vi "Query Sweep Mode.vi"(8 "error in (no error)":errorcluster, 10 "Channel (0: Channel 1)":T2 items=["Channel 1", "Channel 2"], 11 "VISA resource name":refnum<visa-resource-name>) -> (0 "error out":errorcluster, 1 "Sweep mode (auto)":T1, 3 "VISA resource name out":refnum<visa-resource-name>)   [LabVIEW 2009, in "Tektronix AFG 3000 Series.lvlib"]
doc: "Queries the sweep mode of a Tektronix AFG 3000 series function generator; returns either auto or manual. In auto mode the AFG sweeps continuously; in manual mode, it sweeps once each time it gets a trigger."
uses:
  Tektronix AFG 3000 Series.lvlib
  controls.llb/Channel.ctl
  controls.llb/Sweep Mode.ctl
  <vilib>/Utility/error.llb/DialogType.ctl
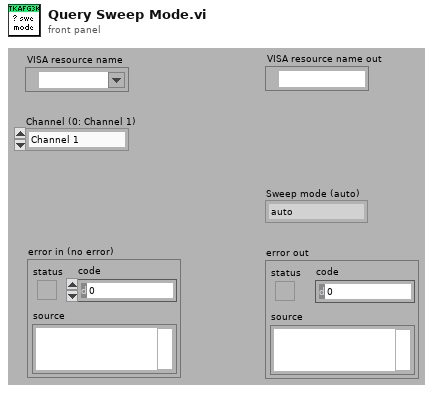
[diagram p1: front panel]
types:
  T1 = typedef "Sweep Mode.ctl" = enum16{"auto", "manual/triggered"}
  T2 = typedef "Channel.ctl" = u16
  T3 = typedef "DialogType.ctl" = u16
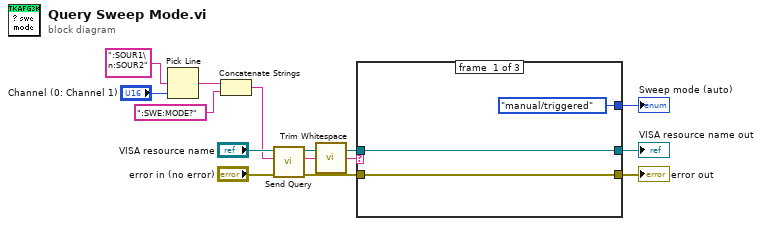
[diagram p0: block diagram]
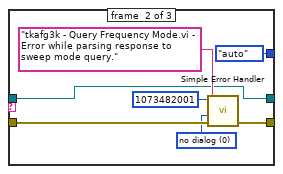
[diagram p2: hidden frame]
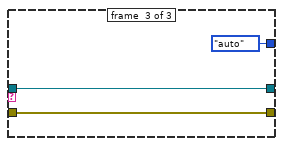
[diagram p3: hidden frame]
diagram:
  n1 = Pick Line(multi-line string=":SOUR1\n:SOUR2", line index="Channel (0: Channel 1)") -> (output string=w11:string)  [unwired: 1 out]
  n2 = Concatenate Strings(w11, ":SWE:MODE?" ("format string")) -> (w10:string)
  n3 = call "Send Query.vi"("error in (no error)"="error in (no error)", "write buffer"=w10, "VISA resource name"="VISA resource name") -> ("error out"=w7:errorcluster, "read buffer"=w3:string, "VISA resource name out"=w6:refnum<visa-resource-name>)  [unwired: 1 in, 5 out]
  n4 = call <vilib>:"Trim Whitespace.vi"("string"=w3) -> ("trimmed string"=w2:string)  [unwired: 1 in]
  n5 = case shown="Default" w2 {
    tunnel: [Sweep_Mode."manual/triggered" ("Sweep mode (auto) 2") Sweep_Mode."auto" ("Sweep mode (auto) 2") Sweep_Mode."auto" ("Sweep mode (auto) 2")] -> w1
    tunnel: w7 -> [w16 w24 w26]
    tunnel: w6 -> [w17 w19 w27]
    tunnel: [w17 w19 w27] -> w5
    tunnel: [w16 w23 w26] -> w4
    frame #0 {
    }
    frame #1 {
      w22 = T3 0 items=["no dialog", "OK message", "continue or stop message", "OK message + warnings", "continue/stop + warnings"] ("type of dialog (OK msg:1)")
      n6 = call <vilib>:"Simple Error Handler.vi"("error code (no error:0)"=1073482001, "error source (\" \")"="tkafg3k - Query Frequency Mode.vi - Error while parsing response to sweep mode query." ("error source (\" \")"), "type of dialog (OK msg:1)"=w22, "error in (no error)"=w24) -> ("error out"=w23:errorcluster)  [unwired: 5 out]
    }
    frame #2 {
    }
  }
  "error out" <- w4
  "VISA resource name out" <- w5
  "Sweep mode (auto)" <- w1
